vi "myRIO_BRig_RT_dataTrial_IallReward_R.vi"() -> (2 "output_I_allReward_R":i32)   [LabVIEW 2014]
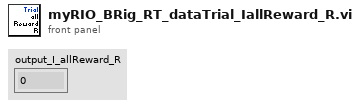
[diagram p1: front panel]
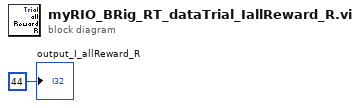
[diagram p0: block diagram]
diagram:
  "output_I_allReward_R" <- 44 ("output_iBlock")
